vi "SCT Have Attrs Changed.vi"(1 "Attrib Changes":T2, 2 "Attribs":T1) -> (0 "Boolean":bool)   [LabVIEW 2016]
uses:
  <resource>/dialog/variable/SCT Attribute Changes.ctl
  <vilib>/variable/Attribs.ctl
  <vilib>/variable/NI_Variable.lvlib
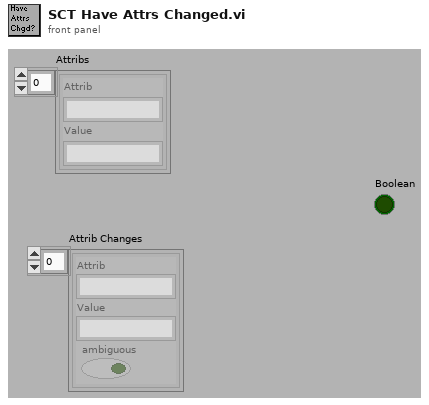
[diagram p1: front panel]
types:
  T1 = typedef "NI_Variable.lvlib/Attribs.ctl" = cluster{"Attrib":string, "Value":string}[]
  T2 = typedef "SCT Attribute Changes.ctl" = cluster{"Attrib":string, "Value":string, "ambiguous":bool}[]
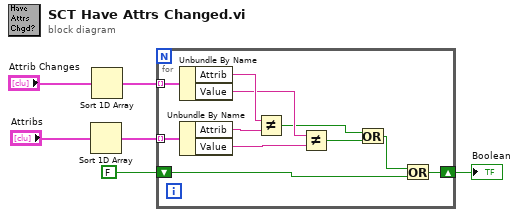
[diagram p0: block diagram]
diagram:
  n1 = Sort 1D Array(array="Attribs") -> (sorted array=w3:T1)
  n2 = Sort 1D Array(array="Attrib Changes") -> (sorted array=w4:T2)
  n3 = for {
    tunnel: w4 -> [w17] mode=indexing
    tunnel: w3 -> [w16] mode=indexing
    shift-right: [w9] -> w1
    shift-left: FALSE -> [w8]
    n4 = Unbundle By Name(w17) -> ("Attrib"=w14:string, "Value"=w12:string)
    n5 = Unbundle By Name(w16) -> ("Attrib"=w15:string, "Value"=w13:string)
    n6 = Not Equal?(x=w14, y=w15) -> (x != y?=w10:bool)
    n7 = Not Equal?(x=w12, y=w13) -> (x != y?=w11:bool)
    n8 = Or(x=w10, y=w11) -> (x .or. y?=w7:bool)
    n9 = Or(x=w7, y=w8) -> (x .or. y?=w9:bool)
  }
  "Boolean" <- w1
